vi "flatten message.vi"(8 "error in":errorcluster, 11 "data message":refnum<class "communicator message.lvclass">) -> (0 "error out":errorcluster, 3 "data":string)   [LabVIEW 2015, in "TCP server.lvclass"]
uses:
  TCP server.lvclass
  message/communicator message.lvclass
  message/communicator message.lvclass/communicator message.ctl
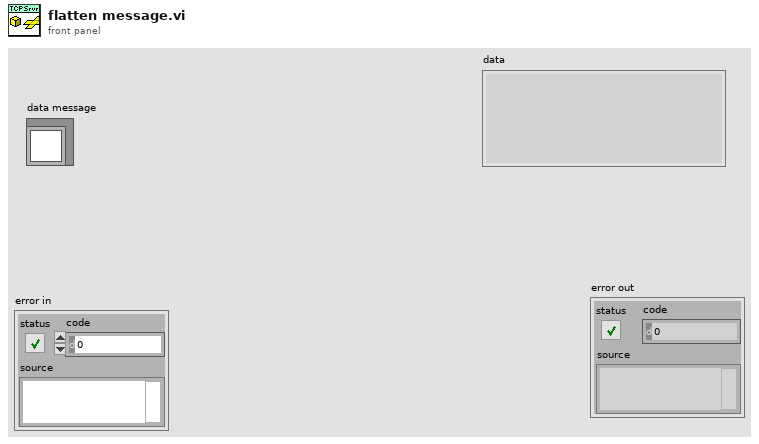
[diagram p1: front panel]
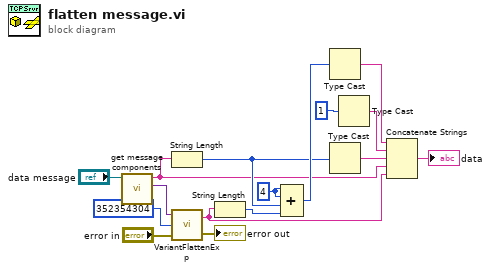
[diagram p0: block diagram]
diagram:
  w8 = 4 ("length (rest)")
  n1 = call "get message components.vi"("message"="data message") -> ("data"=w2:variant, "ID"=w3:string)  [unwired: 9 in]
  n2 = String Length(string=w3) -> (length=w7:i32)
  n3 = call <vilib>:"VariantFlattenExp.vi"("error in (no error)"="error in", "version"=u32 352354304, "variant"=w2) -> ("error out"=→"error out":errorcluster, "data string"=w6:string)
  n4 = String Length(string=w6) -> (length=w5:i32)
  n5 = Compound Arithmetic op=ADD(w8, w8, w7, w5) -> (w10:i32)
  n6 = Type Cast(x=w10) -> (*(type *) &x=w9:string)  [unwired: 1 in]
  n7 = Type Cast(x=w7) -> (*(type *) &x=w11:string)  [unwired: 1 in]
  n8 = Type Cast(x=1 ("length (rest)")) -> (*(type *) &x=w15:string)  [unwired: 1 in]
  n9 = Concatenate Strings(w9, w15, w11, w3, w6) -> (→"data":string)
